vi "opencvSegmentTestLL2.vi"() -> ()   [LabVIEW 2017]
uses:
  <vilib>/Analysis/baseanly.llb/Mean (DBL).vi
  opencvSegmentConvertCoordinates-singleFrame.vi
  <vilib>/Analysis/NI_AALBase.lvlib
panel:
  in  "threshold":sgl=600.0
  out "mean":dbl format="%0.9f"
  out "XY Graph":cluster{dbl[], dbl[]}(graph)
  out "Intensity Graph 3":u16[][](graph)
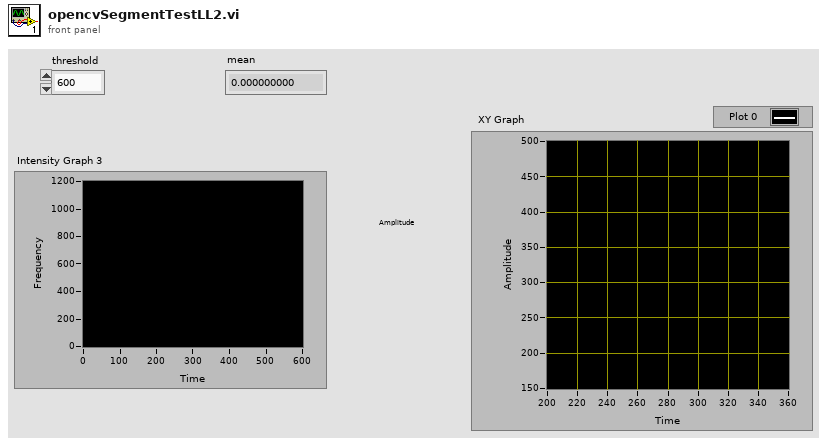
[diagram p1: front panel]
types:
  T1 = enum16{"big-endian, network order", "native, host order", "little-endian"}
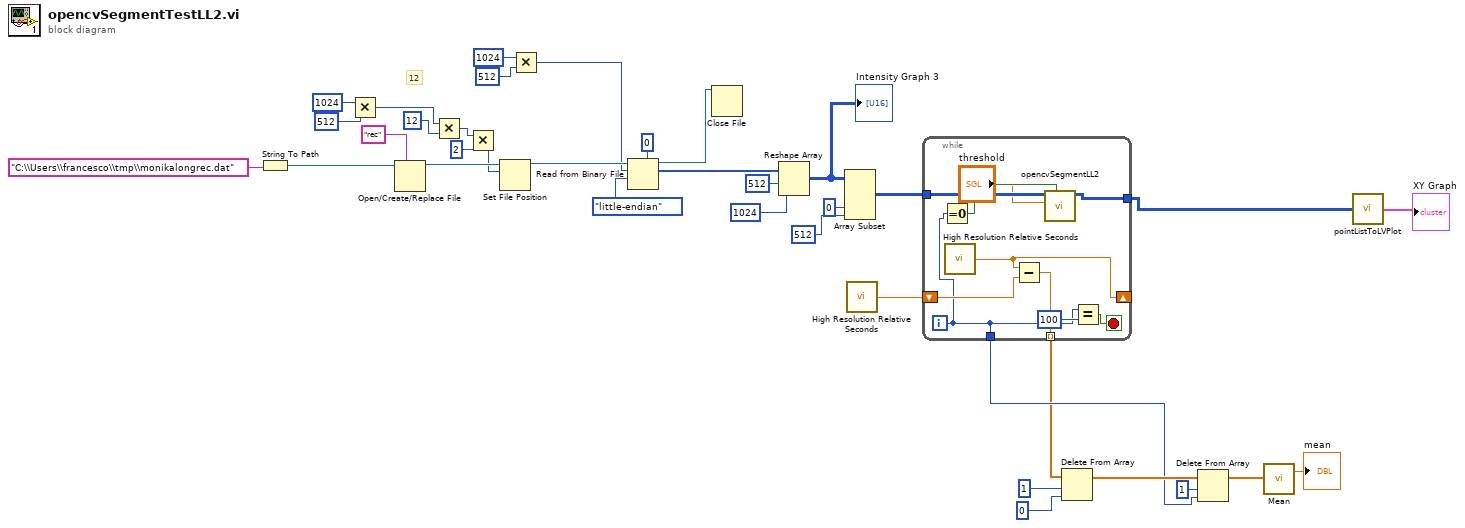
[diagram p0: block diagram]
diagram:
  # "12"
  n1 = String To Path(string="C:\\Users\\francesco\\tmp\\monikalongrec.dat") -> (path=w22:path)
  n2 = Multiply(x=i64 1024, y=i64 512) -> (x*y=w28:i64)
  n3 = Open/Create/Replace File(file path (use dialog)=w22, prompt="rec") -> (refnum out=w29:refnum<file>)  [unwired: 4 in, 2 out]
  n4 = Multiply(x=w28, y=i64 12) -> (x*y=w20:i64)
  n5 = Multiply(x=w20, y=i64 2) -> (x*y=w18:i64)
  n6 = Set File Position(offset (in bytes) (0)=w18, refnum=w29) -> (refnum out=w26:refnum<file>)  [unwired: 2 in, 1 out]
  n7 = Multiply(x=1024, y=512) -> (x*y=w16:i32)
  n8 = Read from Binary File(5:u16 0, 9:T1."little-endian" ("byte order (0:big-endian, network order)"), 10:w16, 11:w26) -> (2:w30:u16[], 3:w21:refnum<file>)  [unwired: 2 in, 2 out]
  n9 = Close File(refnum=w21) -> ()  [unwired: 1 in, 2 out]
  n10 = Reshape Array(w30, 512 ("dimension size"), 1024 ("dimension size")) -> (w14:u16[][])
  "Intensity Graph 3" <- w14
  n11 = Array Subset(array=w14, index (col)=0 ("index"), length (col)=512 ("length")) -> (w11:u16[][])  [unwired: 2 in]
  n12 = call <vilib>:"High Resolution Relative Seconds.vi"() -> ("relative seconds"=w10:dbl)
  n13 = while {
    tunnel: w11 -> [w46]
    tunnel: [w45] -> w1
    shift-right: [w43] -> _
    shift-left: w10 -> [w44]
    tunnel: [w42] -> w3 mode=indexing
    tunnel: [w40] -> w4
    i -> [w40]
    stop <- w39 stop-if-true
    n14 = Equal To 0?(x=w40) -> (x = 0?=w38:bool)
    n15 = call <vilib>:"High Resolution Relative Seconds.vi"() -> ("relative seconds"=w43:dbl)
    n16 = Subtract(x=w43, y=w44) -> (x-y=w42:dbl)
    n17 = call "opencvSegmentLL2.vi"("allocate"=w38, "threshold"="threshold", "ImgIn"=w46) -> ("NeuronYX"=w45:u16[][])  [unwired: 7 in, 1 out]
    n18 = Equal?(x=w40, y=100) -> (x = y?=w39:bool)
  }
  n19 = Delete From Array(array=w3, length=1, index=0) -> (array with subset deleted=w8:dbl[])  [unwired: 1 out]
  n20 = Delete From Array(array=w8, length=1, index=w4) -> (array with subset deleted=w2:dbl[])  [unwired: 1 out]
  n21 = call-poly <vilib>:"Mean.vi"("X"=w2) -> ("mean"=→"mean":dbl)  [unwired: 1 out]
  n22 = call "pointListToLVPlot.vi"("XY[N,d]"=w1) -> ("LV plot"=→"XY Graph":cluster{dbl[], dbl[]})
